vi "Format Instrument String Response.vi"(6 "Response Parameters":T1, 8 "error in (no error)":errorcluster, 9 "Data Lookup in":variant, 10 "Data":dbl[](array[numeric]), 11 "Response":string) -> (0 "error out":errorcluster, 1 "Data Lookup out":variant, 2 "Data out":dbl[](array[numeric]))   [LabVIEW 2019, in "Instrument Addon Engine.lvlib"]
uses:
  Instrument Addon Engine.lvlib
  Addon Shared/Types/Response RT Configuration Cluster.ctl
  Addon Shared/Types/Response Parameters.ctl
  Addon Shared/Types/Linked Channel Cluster.ctl
  Addon Shared/Types/Response Wait Type.ctl
  Addon Shared/Types/Data RT Configuration Cluster.ctl
  Addon Shared/Types/Data Parameters.ctl
  Addon Shared/Types/Protocol Data Type.ctl
  Addon Shared/Types/Data Channel Type.ctl
  Addon Shared/Types/Type Cast Type.ctl
  Addon Shared/Types/Endian.ctl
  Addon Shared/Instrument Addon Shared.lvlib
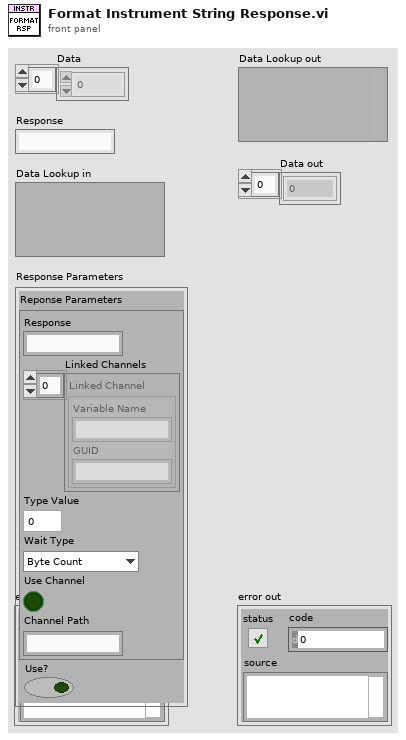
[diagram p1: front panel]
types:
  T1 = typedef "Instrument Addon Shared.lvlib/Response RT Configuration Cluster.ctl" = cluster{"Reponse Parameters":T2, "Use?":bool}
  T2 = typedef "Instrument Addon Shared.lvlib/Response Parameters.ctl" = cluster{"Response":string, "Linked Channels":T3[], "Type Value":dbl, "Wait Type":T4, "Use Channel":bool, "Channel Path":string}
  T3 = typedef "Instrument Addon Shared.lvlib/Linked Channel Cluster.ctl" = cluster{"Variable Name":string, "GUID":string}
  T4 = typedef "Instrument Addon Shared.lvlib/Response Wait Type.ctl" = enum16{"Byte Count", "Wait sec"}
  T5 = typedef "Instrument Addon Shared.lvlib/Data RT Configuration Cluster.ctl" = cluster{"Data Parameters":T6, "Data Index":i32, "Data Length":i32}
  T6 = typedef "Instrument Addon Shared.lvlib/Data Parameters.ctl" = cluster{"Data Type":T7, "Channel Type":T8, "Format String":string, "Expected String":string, "Type":T9, "List":string[], "Delimiter":string, "Endian":T10}
  T7 = typedef "Instrument Addon Shared.lvlib/Protocol Data Type.ctl" = enum16{"Single Channel", "Array"}
  T8 = typedef "Instrument Addon Shared.lvlib/Data Channel Type.ctl" = enum16{"Format", "Comparison", "Type Cast", "Enumerated List"}
  T9 = typedef "Instrument Addon Shared.lvlib/Type Cast Type.ctl" = enum16{"DBL", "SGL", "U64", "U32", "U16", "U8", "I64", "I32", "I16", "I8"}
  T10 = typedef "Instrument Addon Shared.lvlib/Endian.ctl" = enum16{"Native", "Little", "Big"}
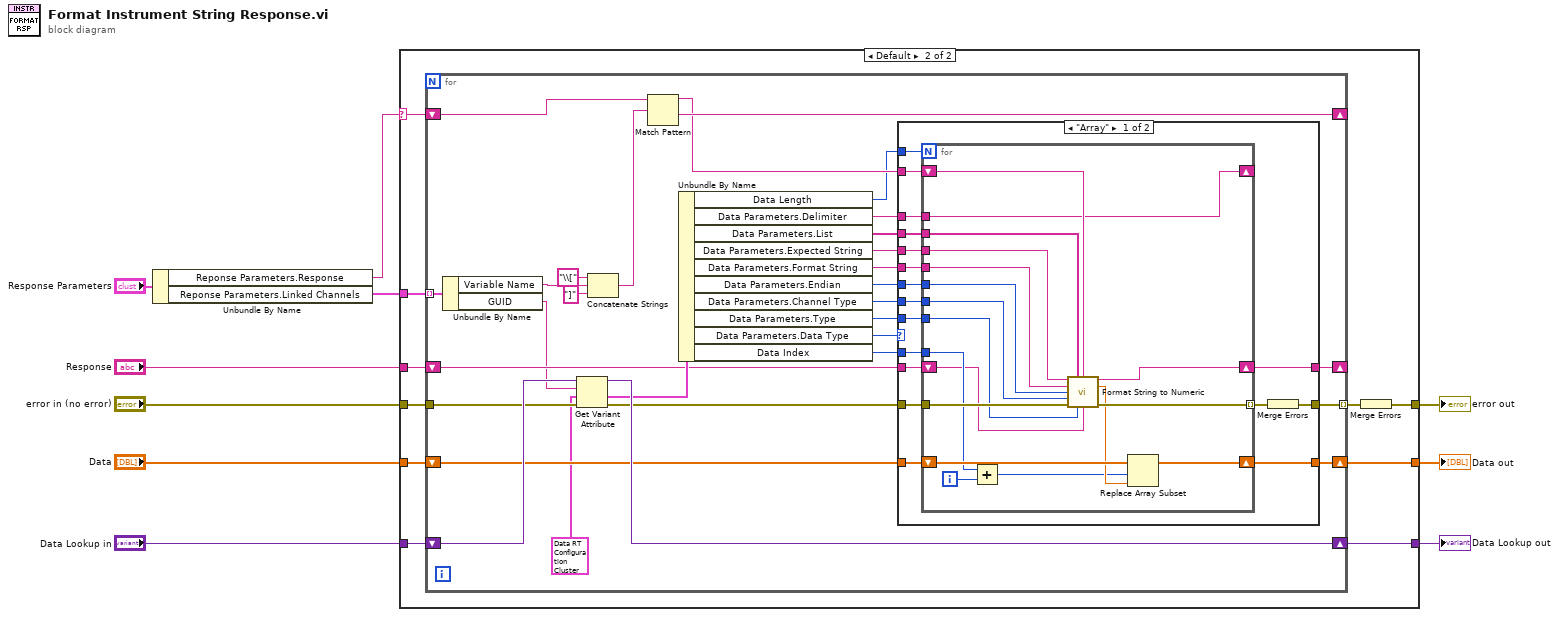
[diagram p0: block diagram]
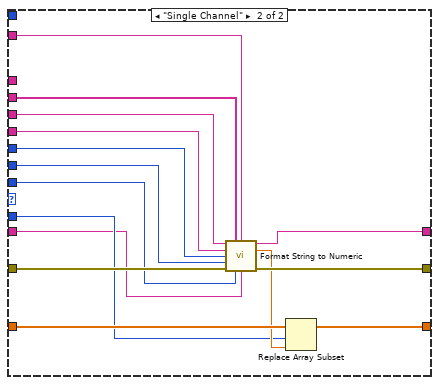
[diagram p3: hidden frame]
diagram:
  n1 = Unbundle By Name("Response Parameters") -> ("Reponse Parameters.Response"=w2:string, "Reponse Parameters.Linked Channels"=w5:T3[])
  n2 = case shown="Default" w2 {
    selector: w2 -> [_ w15]
    tunnel: [w13 w14] -> w10
    tunnel: "error in (no error)" -> [w13 w22]
    tunnel: "Response" -> [_ w21]
    tunnel: [w11 w20] -> w8
    tunnel: [w12 w19] -> w7
    tunnel: "Data" -> [w11 w18]
    tunnel: w5 -> [_ w17]
    tunnel: "Data Lookup in" -> [w12 w16]
    frame "" {
    }
    frame Default {
      n3 = for {
        tunnel: [w48] -> _ mode=indexing
        shift-right: [w51] -> w19
        shift-left: w16 -> [w53]
        shift-right: [w35] -> _
        shift-left: w15 -> [w39]
        tunnel: w17 -> [w48] mode=indexing
        shift-right: [w46] -> w20
        shift-left: w18 -> [w49]
        shift-right: [w43] -> _
        shift-left: w21 -> [w45]
        tunnel: w22 -> [w52]
        tunnel: [w36] -> w23 mode=indexing
        n4 = Unbundle By Name(w48) -> ("Variable Name"=w40:string, "GUID"=w33:string)
        n5 = Get Variant Attribute(Variant=w53, name=w33, default value (empty Variant)=T5 {"Data Parameters"={"Data Type"=enum."Single Channel", "Channel Type"=enum."Format", "Format String"="", "Expected String"="", "Type"=enum."DBL", "List"=[], "Delimiter"="", "Endian"=enum."Native"}, "Data Index"=0, "Data Length"=0}, error in=w52) -> (duplicate Variant=w51:variant, value=w50:T5, error out=w37:errorcluster)  [unwired: 1 out]
        n6 = Concatenate Strings("\\[" ("string"), w40, "]" ("string")) -> (w31:string)
        n7 = Match Pattern(string=w39, regular expression=w31) -> (before substring=w34:string, after substring=w35:string)  [unwired: 1 in, 2 out]
        n8 = Unbundle By Name(w50) -> ("Data Length"=w28:i32, "Data Parameters.Delimiter"=w27:string, "Data Parameters.List"=w29:string[], "Data Parameters.Expected String"=w32:string, "Data Parameters.Format String"=w38:string, "Data Parameters.Endian"=w24:T10, "Data Parameters.Channel Type"=w44:T8, "Data Parameters.Type"=w30:T9, "Data Parameters.Data Type"=w26:T7, "Data Index"=w25:i32)
        n9 = case shown="\"Array\"" w26 {
          tunnel: w49 -> [w70 w103]
          tunnel: [w69 w102] -> w46
          tunnel: w45 -> [w68 w90]
          tunnel: w44 -> [w67 w101]
          tunnel: [w66 w92] -> w43
          tunnel: w38 -> [w65 w100]
          tunnel: w37 -> [w64 w99]
          tunnel: [w56 w98] -> w36
          tunnel: w34 -> [w63 w91]
          tunnel: w25 -> [w62 w93]
          tunnel: w32 -> [w61 w97]
          tunnel: w30 -> [w60 w96]
          tunnel: w29 -> [w59 w95]
          tunnel: w28 -> [w58 _]
          tunnel: w27 -> [w55 _]
          tunnel: w24 -> [w54 w89]
          frame "Array" {
            n10 = for {
              N: w58 -> [_]
              tunnel: w67 -> [w72]
              tunnel: w65 -> [w86]
              tunnel: w62 -> [w83]
              tunnel: w61 -> [w82]
              tunnel: w60 -> [w80]
              tunnel: w59 -> [w79]
              shift-right: [w87] -> w69
              shift-left: w70 -> [w88]
              shift-right: [w76] -> w66
              shift-left: w68 -> [w75]
              tunnel: w64 -> [w85]
              tunnel: [w84] -> w57 mode=indexing
              shift-right: [w71] -> _
              shift-left: w63 -> [w74]
              tunnel: w55 -> [w71]
              tunnel: w54 -> [w73]
              i -> [w77]
              n11 = Add(x=w83, y=w77) -> (x+y=w78:i32)
              n12 = call "Format String to Numeric.vi"("Expected String"=w82, "Data Parameters.List"=w79, "Ignore String"=w74, "Format String"=w86, "Endian"=w73, "Channel Type"=w72, "error in (no error)"=w85, "Type"=w80, "Response"=w75) -> ("remaining string"=w76:string, "Value"=w81:dbl, "error out"=w84:errorcluster)  [unwired: 4 in]
              n13 = Replace Array Subset(array=w88, new element=w81, index=w78) -> (w87:dbl[])
            }
            n14 = Merge Errors(w57) -> (w56:errorcluster)
          }
          frame "Single Channel" {
            n15 = call "Format String to Numeric.vi"("Expected String"=w97, "Data Parameters.List"=w95, "Ignore String"=w91, "Format String"=w100, "Endian"=w89, "Channel Type"=w101, "error in (no error)"=w99, "Type"=w96, "Response"=w90) -> ("remaining string"=w92:string, "Value"=w94:dbl, "error out"=w98:errorcluster)  [unwired: 4 in]
            n16 = Replace Array Subset(array=w103, new element=w94, index=w93) -> (w102:dbl[])
          }
        }
      }
      n17 = Merge Errors(w23) -> (w14:errorcluster)
    }
  }
  "error out" <- w10
  "Data out" <- w8
  "Data Lookup out" <- w7
